vi "Configure Reference Oscilator.vi"(8 "error in (no error)":errorcluster, 9 "External Frequency (10MHz)":dbl=10000000.0 format="%#.9p", 10 "Frequency Source (Internal)":i32(ring) items=["Internal", "External"], 11 "VISA resource name":refnum<visa-resource-name>) -> (0 "error out":errorcluster, 3 "VISA resource name out":refnum<visa-resource-name>)   [LabVIEW 2020, in "Rohde&Schwarz CMXP Base.lvlib"]
doc: "Selects the reference frequency source to be used.\n\nAttributes:\nRSCMXPBASE_ATTR_SYSTEM_REFERENCE_FREQUENCY_SOURCE\nRSCMXPBASE_ATTR_SYSTEM_REFERENCE_EXTERNAL_FREQUENCY\n\nRemote-control commands:\nSYSTem:BASE:REFerence:FREQuency:SOURce\nSYSTem:BASE:REFerence:FREQuency"
uses:
  <instrlib>/Rohde&Schwarz CMXP Base/Rohde&Schwarz CMXP Base.lvlib
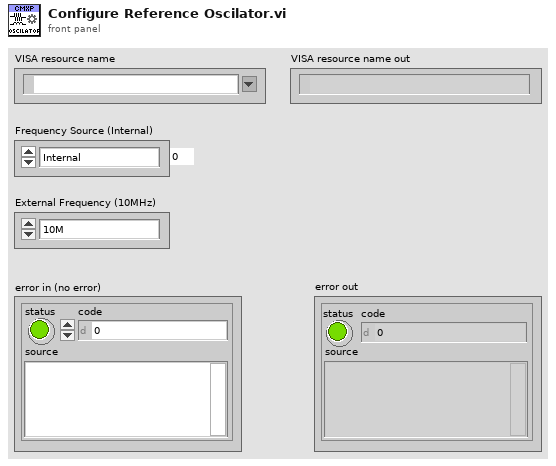
[diagram p1: front panel]
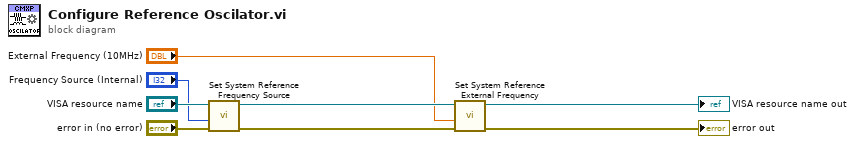
[diagram p0: block diagram]
diagram:
  n1 = call "Set System Reference Frequency Source"("error in (no error)"="error in (no error)", "System Reference Frequency Source (0 - Internal)"="Frequency Source (Internal)", "instrument handle"="VISA resource name") -> ("error out"=w6:errorcluster, "instrument handle out"=w5:refnum<visa-resource-name>)  [unwired: 7 in]
  n2 = call "Set System Reference External Frequency"("error in (no error)"=w6, "System Reference External Frequency (0.0)"="External Frequency (10MHz)", "instrument handle"=w5) -> ("error out"=→"error out":errorcluster, "instrument handle out"=→"VISA resource name out":refnum<visa-resource-name>)  [unwired: 7 in]
